vi "MeanderCtrl_Dynamic,StageRefs.vi"(0 "QueuesRef":T1, 1 "MotionStageRefs":refnum<queue>, 2 "AppsRef":refnum<queue>, 3 "subprog_Ref":refnum<vi>, 7 "Params.":variant, 9 "Laser_Ctrl":bool, 11 "error in":errorcluster, 12 "HighSpeed":dbl=5.0, 13 "LowSpeed":dbl=0.1) -> (6 "Interupted":bool, 15 "error out":errorcluster)   [LabVIEW 2013]
uses:
  ControlDef/QueueRefs.ctl
  ControlDef/LaserCtrl_Method.ctl
  ControlDef/States-AToF.ctl
  <instrlib>/AnalogDiscSDKLv/VIs/DWF_CtrlQueue.ctl
  <instrlib>/AnalogDiscSDKLv/VIs/DWF_State.ctl
  <instrlib>/ESP300/Public/Data/ESP300_State.ctl
  <instrlib>/DG535/Command/DG535_States.ctl
  Hardware/BNC(QuantumComposers)/BNC_States.ctl
  Hardware/FemtoLaser(Legacy)/Laser_Status.ctl
  Hardware/DAQmx(Legacy)/DAQmx_Status.ctl
  ControlDef/Signal.ctl
  ProcessMethods/SignalAverager/ProcessStates.ctl
  Files/WriterState.ctl
  Files/Signal_Segment.ctl
  ControlDef/ProcessingMode.ctl
  Hardware/EPM2000(Legacy)/EPM2K_Status.ctl
  <instrlib>/AnalogDiscSDKLv/VIs/DWF_Signal.ctl
  Apps_static/MeanderLoopState.ctl
  Apps_static/ScanParams_SingleLine.ctl
  <instrlib>/ESP300/Public/Data/ESP30x_Data.ctl
  <vilib>/Utility/error.llb/DialogType.ctl
  ControlDef/PauseMeander.vi
  <instrlib>/ESP300/ESP300.lvlib
  <instrlib>/DG535/SRS_DG535_Lib.lvlib
  <userlib>/Utility/ErrorLog_lib.lvlib
  <instrlib>/AnalogDiscSDKLv/AnalogDiscSDKLv.lvlib
panel:
  in  "TotalScan":i32
  out "timed out?":bool
  out "Core_iter.":i32
  out "Scanned Lines":i32
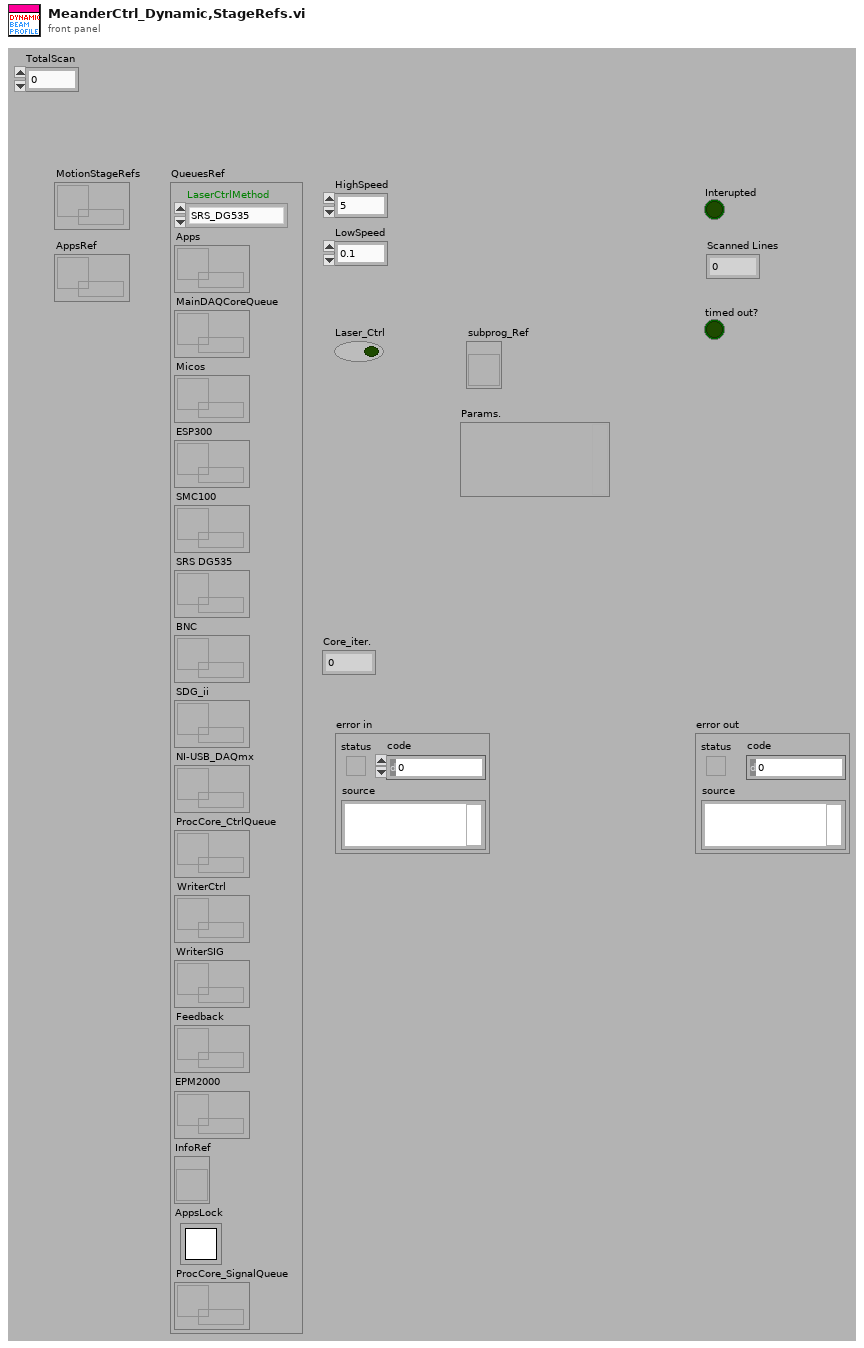
[diagram p1: front panel]
types:
  T1 = typedef "QueueRefs.ctl" = cluster{"LaserCtrlMethod":T2, "Apps":refnum<queue>, "MainDAQCoreQueue":refnum<queue>, "Micos":refnum<queue>, "ESP300":refnum<queue>, "SMC100":refnum<queue>, "SRS DG535":refnum<queue>, "BNC":refnum<queue>, "SDG_ii":refnum<queue>, "NI-USB_DAQmx":refnum<queue>, "ProcCore_CtrlQueue":refnum<queue>, "WriterCtrl":refnum<queue>, "WriterSIG":refnum<queue>, "Feedback":refnum<queue>, "EPM2000":refnum<queue>, "InfoRef":refnum<vi>, "AppsLock":T3, "ProcCore_SignalQueue":refnum<queue>}
  T2 = typedef "LaserCtrl_Method.ctl" = enum16{"SRS_DG535", "BNC", "SDG_II"}
  T3 = typedef "Semaphore RefNum" = refnum<k1>
  T4 = typedef "States-AToF.ctl" = enum16{"Initialize", "Idle", "CalcMzArray", "Meander_SGL_MCS", "Meander_MCS", "CleanSurface", "Meander_Npt", "Meander_SGL_Npt", "KnifeEdgeExpt", "KnifeEdgeExpt_Npt", "Imaging_Micos", "Imaging_ESP", "DepthProfiling", "Set_2PulseDelay", "DelayScan", "PeakSearch", "ExportOrigin", "Save Settings", "Load Settings", "Save as Default", "Load Default", "EnergyCalibration", "Quit", "Interrupted_Stop", "Quit_SubProgram", "StepMove_Joystick", "ContMove_Joystick", "Stop_Joystick", "Check_AppsLock", "Return_Status", "DepthProfile_RT", "UpdateInstruStates", "InstruOptimizer_static", "InstruOptimizer_dynamic", "DepthProfiling(3D)"}
  T5 = typedef "ScanParams_SingleLine.ctl" = cluster{"Line Start":dbl[], "Line End":dbl[], "HighSpeed":dbl, "ScanSpeed":dbl, "KeepStill(ms)":u32, "InstruParams":dbl[]}
  T6 = typedef "MeanderLoopState.ctl" = enum16{"Pre-Start", "Send-loginfo", "SetHighVelocity", "MoveToLineStart", "SetSecondaryParams", "WaitStartReady", "UpdateStartPosition", "StartOfLine", "SetLowVelocity", "MoveToLineEnd", "StartLaser_move", "WaitScanFinish", "StartLaser_still", "KeepStill", "StopLaser", "EndOfLine", "CheckPause", "Exit", "RestoreVelocity", "Pause", "Quit"}
  T7 = typedef "ESP300.lvlib/ESP300_State.ctl" = cluster{"State":enum16{"Initialize", "SetDefaultConfig", "Close", "Quit", "Identify", "MoveAbs", "MoveAbs_all", "MoveRel", "MoveRel_all", "STOP", "Origin/Home", "WaitStop", "QueryStatus", "UpdateXPos", "UpdateAll", "SetVelocity", "SetAcceleration", "ClearErr", "LogMessage", "MotorEnable(1)", "EnableAxis", "JoyStick", "GetVelocity", "GetAcceleration", "SendCmd", "SetSoftLimits", "Beep", "_SettingReturn", "SoftReset"}, "Params.":variant}
  T8 = typedef "ESP300.lvlib/ESP30x_Data.ctl" = cluster{"Position":dbl[], "Velocity":dbl[], "Acceleration":dbl[], "Moving":bool, "Simulation":bool, "tickcount_mov":u32, "tickcount_pos":u32, "NumOfAxis":i32, "Initialized":bool, "CommPort":refnum<visa-resource-name>, "Range":dbl[][], "Serial Configuration":cluster{"Baud Rate":u32, "Parity":u16, "Data Bits":u16, "Stop Bits":u16, "Flow Control":u16}, "MotorDisabled":refnum<vi>}
  T9 = typedef "Signal.ctl" = cluster{"Command":T10, "Params":variant}
  T10 = typedef "ProcessStates.ctl" = enum16{"Initialize", "Normal", "Display", "Write2Buffer", "CalcMzArray", "StartSave", "StopSave", "ConfigChanged", "EndOfLine", "SetFilterParams", "SetGraphsEnable", "SetAcquisitionParams", "ChangeDisplayIncrement", "ChangeRepRate", "SetWriterRef", "Quit", "StartOfLine"}
  T11 = typedef "Laser_Status.ctl" = cluster{"State":enum16{"Initialize", "Idle/Update", "Configure", "Turn On", "Tun OFF", "Continuous", "Single Shot", "ManualTrigger", "Close", "Quit"}, "Parameter":dbl}
  T12 = typedef "BNC_States.ctl" = cluster{"State":enum16{"Initialize", "Set System", "Set C-Input", "Set C-Mode", "Set C-Output", "Set C-Enable", "Manl_Trig", "Run", "Stop", "Query C Number", "Close", "Quit"}, "Para.":variant}
  T13 = typedef "SRS_DG535_Lib.lvlib/DG535_States.ctl" = cluster{"State":enum16{"Initialize", "Set Trigger", "Set Output", "Set Delay", "Manl_Trig", "Run", "Stop", "Close", "Quit"}, "Para.":variant}
  T14 = enum16{"Pre-Start", "Send-loginfo", "SetHighVelocity", "MoveToLineStart", "WaitStartReady", "UpdateStartPosition", "StartOfLine", "SetLowVelocity", "MoveToLineEnd", "StartLaser", "WaitScanFinish", "StopLaser", "EndOfLine", "CheckPause", "Exit", "RestoreHighVelocity", "Pause"}
  T15 = cluster{"Line Start[0]":dbl, "Line Start[1]":dbl, "Line Start[2]":dbl}
  T16 = cluster{"Line End[0]":dbl, "Line End[1]":dbl, "Line End[2]":dbl}
  T17 = typedef "DialogType.ctl" = u16
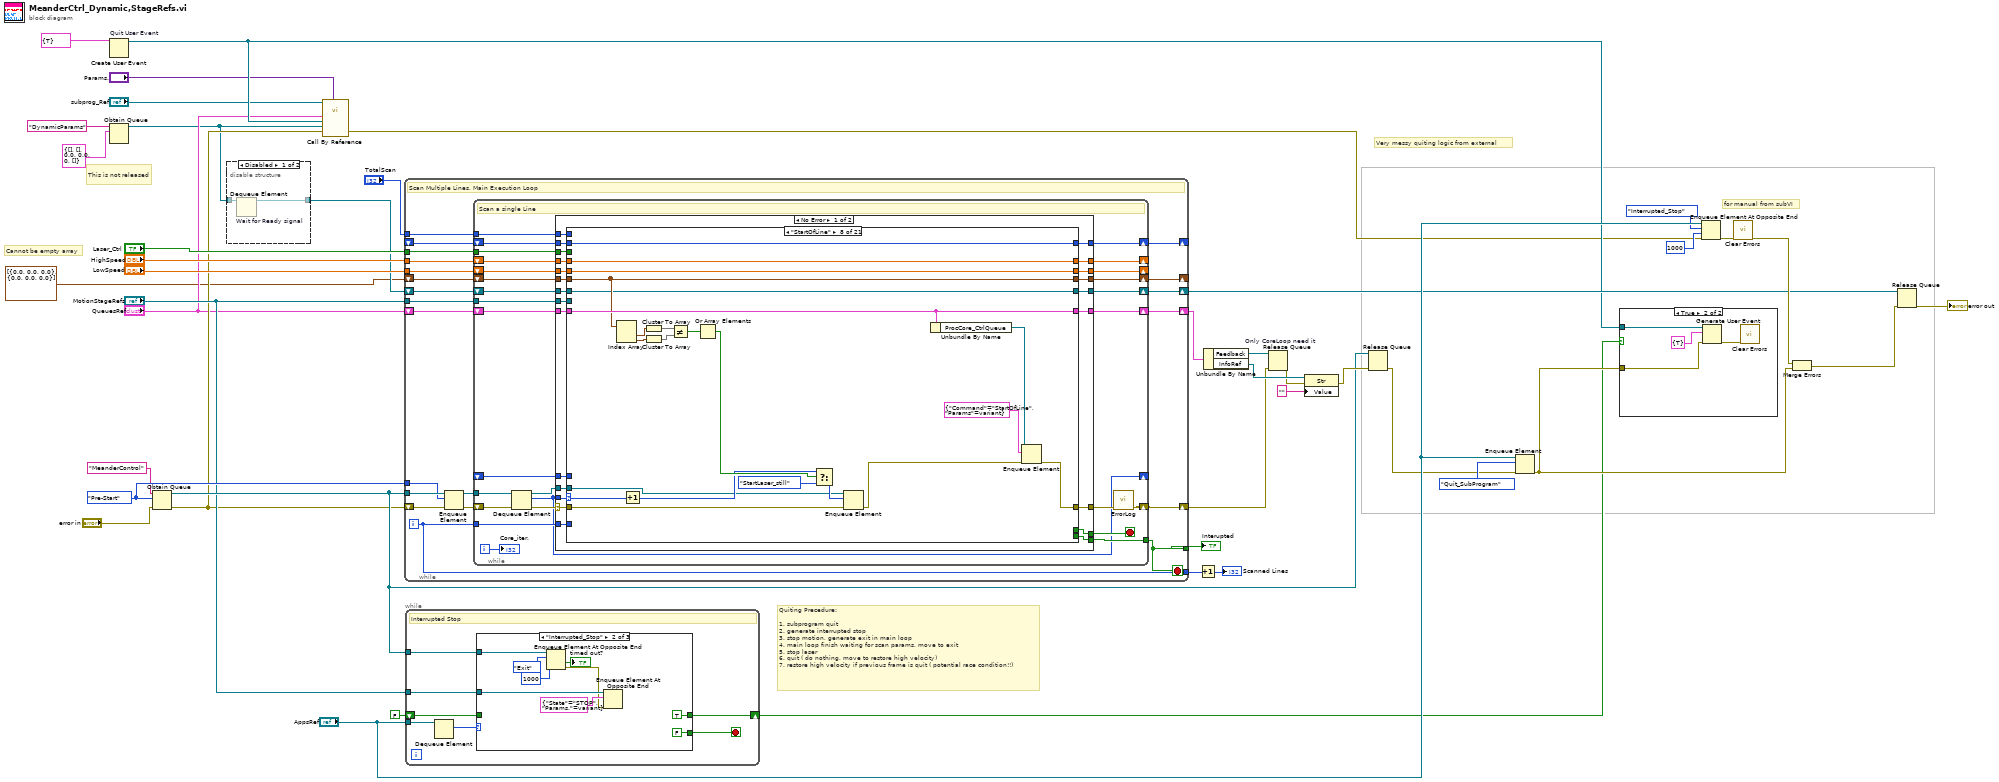
[diagram p0: block diagram]
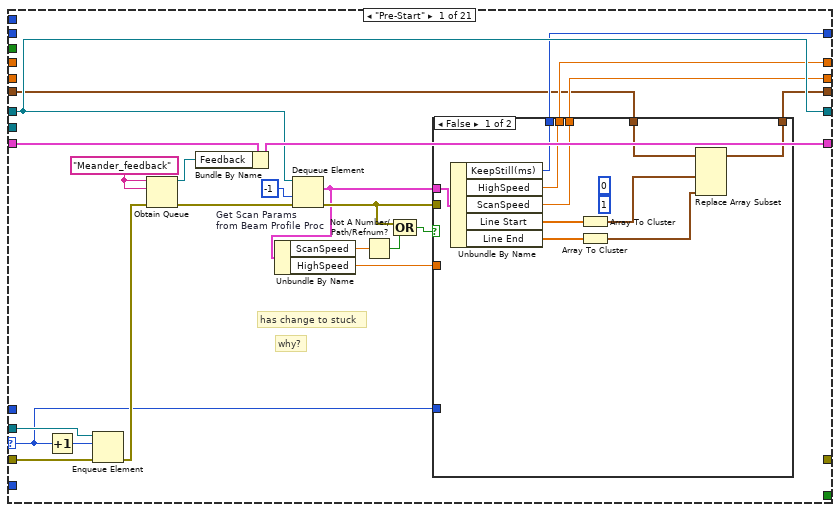
[diagram p2: hidden frame]
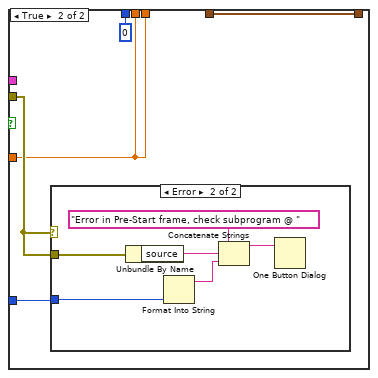
[diagram p3: hidden frame]
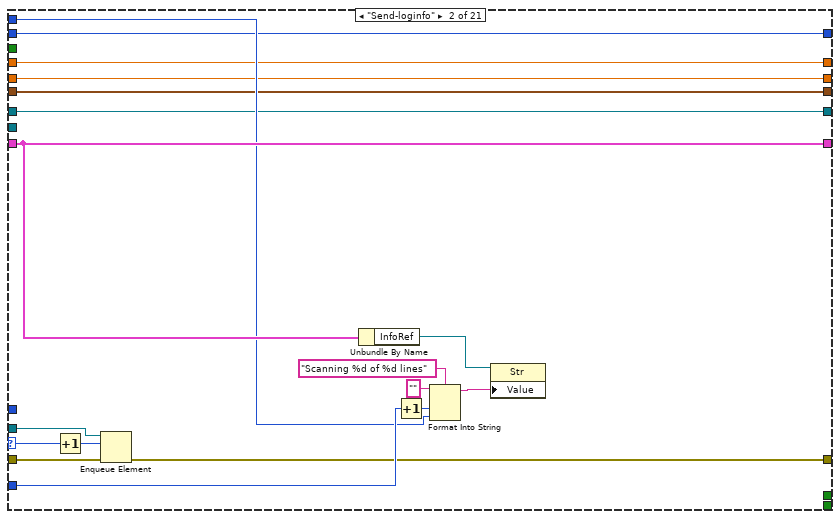
[diagram p5: hidden frame]
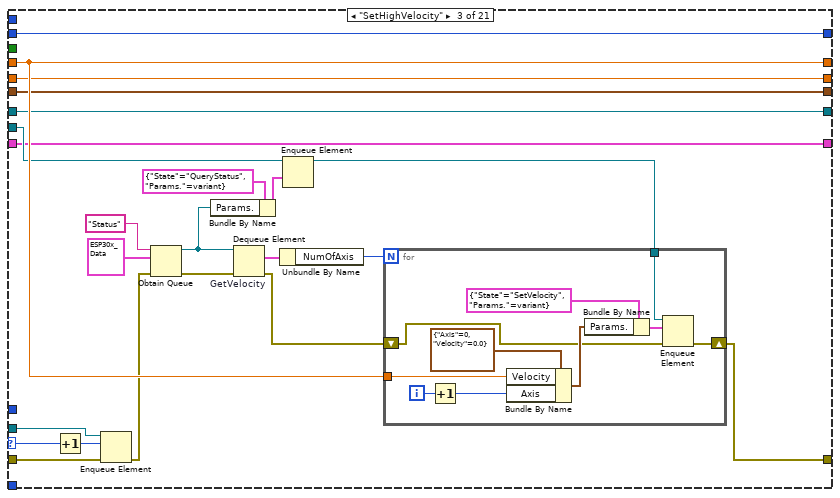
[diagram p6: hidden frame]
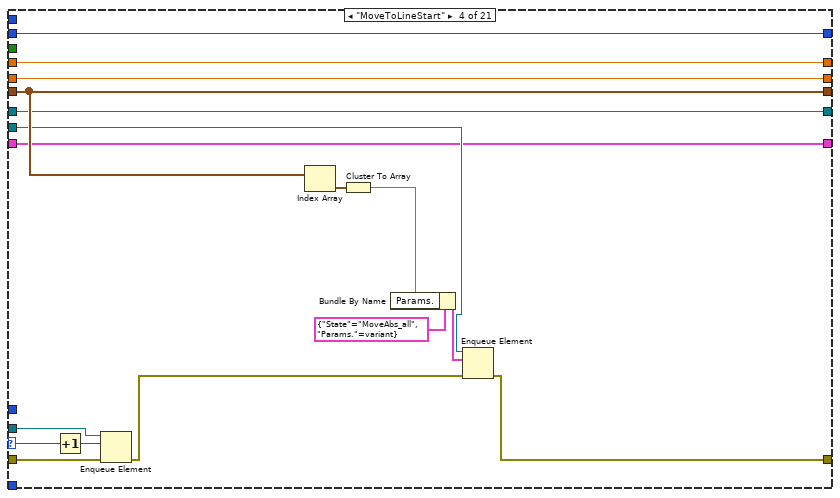
[diagram p7: hidden frame]
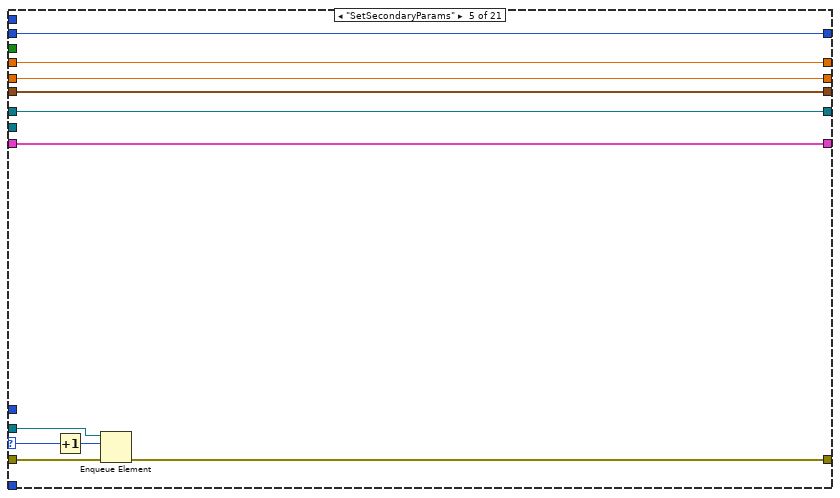
[diagram p8: hidden frame]
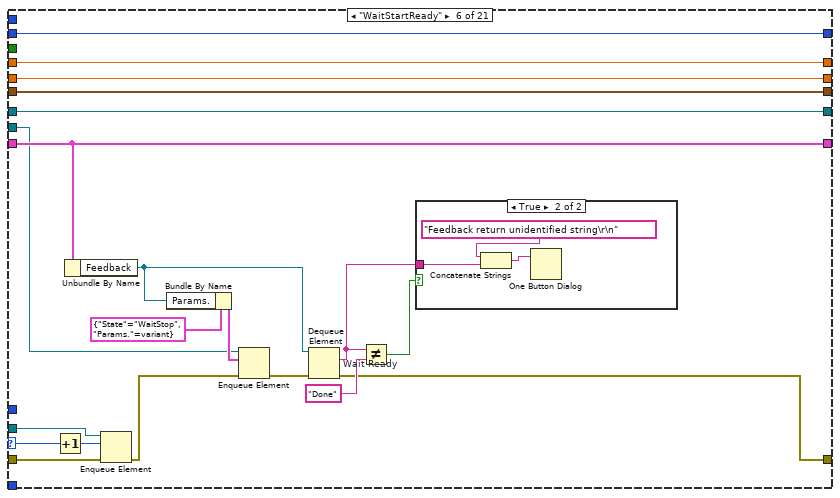
[diagram p9: hidden frame]
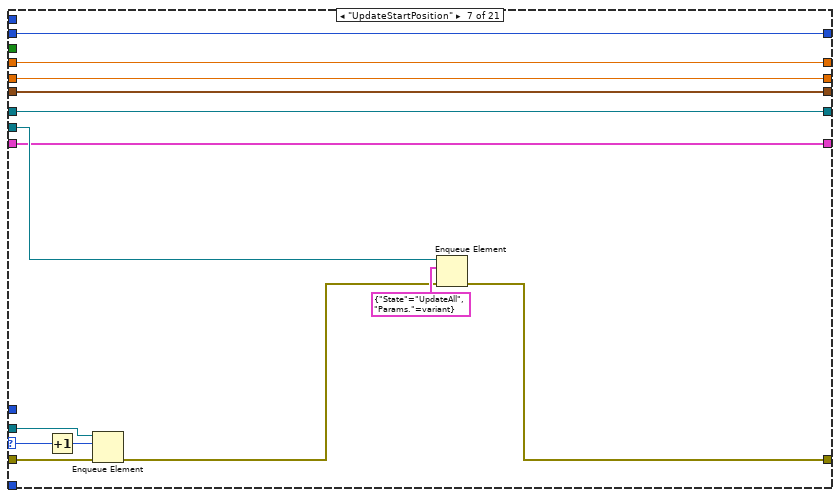
[diagram p11: hidden frame]
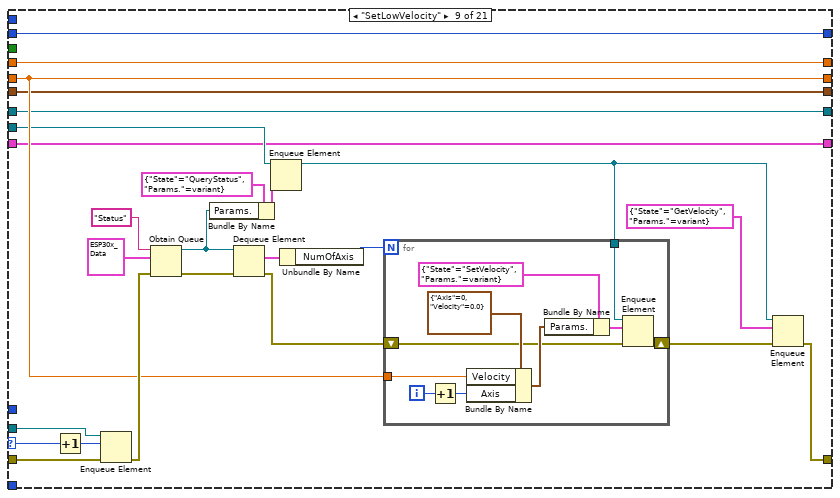
[diagram p12: hidden frame]
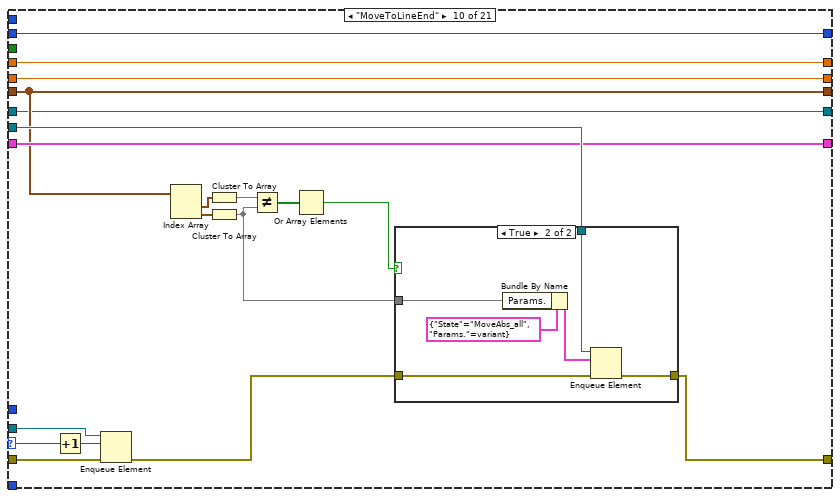
[diagram p13: hidden frame]
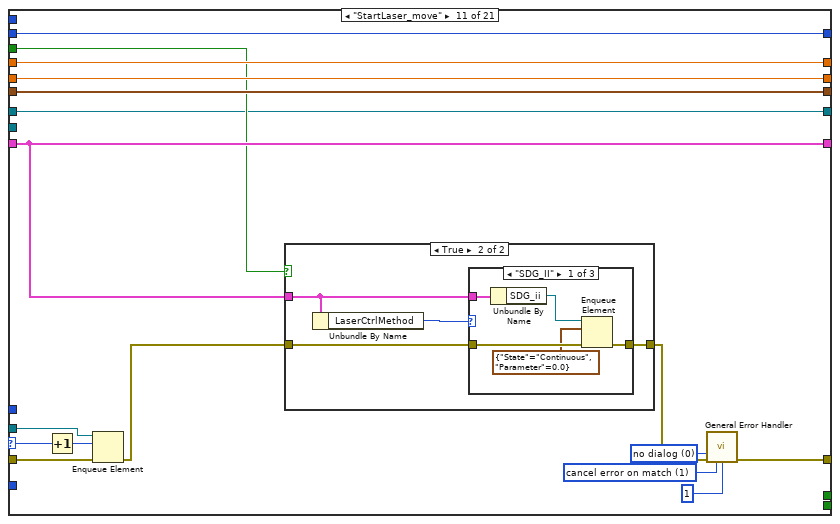
[diagram p15: hidden frame]
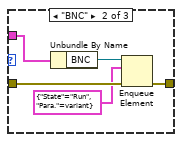
[diagram p17: hidden frame]
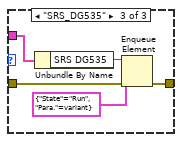
[diagram p18: hidden frame]
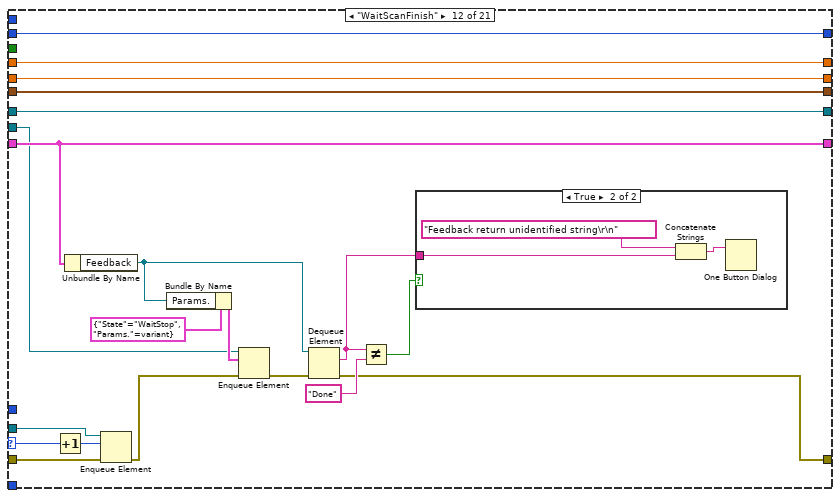
[diagram p19: hidden frame]
diagram:
  w38 = MeanderLoopState."Pre-Start"
  # "Cannot be empty array"
  # "Quiting Precedure:\n\n1. subprogram quit\n2. generate interrupted stop\n3. stop motion, generate exit in main loop\n4. main loop finish waiting for scan params, move to exit \n5. stop laser\n6. quit ( do nothing, move to restore high velocity)\n7. restore high velocity if previous frame is quit ( potential race condition!!)"
  # "Very messy quiting logic from external"
  # "This is not released"
  # "for manual from subVI"
  n1 = Create User Event "Quit User Event"(user event datatype=cluster{"Quit":bool} {"Quit"=TRUE} ("Quit")) -> (user event=w10:refnum<user-event>)  [unwired: 1 in, 1 out]
  n2 = Obtain Queue(name (unnamed)="DynamicParams", element data type=T5 {"Line Start"=[], "Line End"=[], "HighSpeed"=0.0, "ScanSpeed"=0.0, "KeepStill(ms)"=0, "InstruParams"=[]}) -> (queue out=w3:refnum<queue>)  [unwired: 3 in, 2 out]
  n3 = Obtain Queue(name (unnamed)="MeanderControl", element data type=w38, error in (no error)="error in") -> (queue out=w23:refnum<queue>, error out=w9:errorcluster)  [unwired: 2 in, 1 out]
  n4 = disable-structure shown="Disabled" {
    disable-tunnel: w3 -> [w46 w47]
    disable-tunnel: [w45 w47] -> w4
    frame Disabled {
      n5 = Dequeue Element "Wait for Ready signal"(queue=w46) -> (queue out=w45:refnum<queue>)  [unwired: 2 in, 3 out]
    }
    frame Enabled {
    }
  }
  n6 = call-by-ref "?"(reference="subprog_Ref", "Params."="Params.", "error in (no error)"=w9, "Dynamic Params In"=w3, "Quit_UserEvent"=w10, "ControlQueueRef"="QueuesRef") -> ("error out"=w8:errorcluster)  [unwired: 6 in, 3 out]
  n7 = while {
    tunnel: "MotionStageRefs" -> [w67]
    tunnel: w23 -> [w63]
    tunnel: "Laser_Ctrl" -> [w62]
    tunnel: [w61] -> w42
    shift-right: [w60] -> w29
    shift-left: w9 -> [w59]
    tunnel: [w58] -> w39
    tunnel: w38 -> [w56]
    shift-right: [w55] -> w31
    shift-left: "QueuesRef" -> [w66]
    tunnel: "HighSpeed" -> [w64]
    tunnel: "LowSpeed" -> [w65]
    shift-right: [w50] -> w16
    shift-left: w4 -> [w54]
    shift-right: [w49] -> _
    shift-left: _ -> [w53]
    tunnel: "TotalScan" -> [w48]
    shift-right: [w51] -> _
    shift-left: cluster{dbl, dbl, dbl}[] [{0.0, 0.0, 0.0}, {0.0, 0.0, 0.0}] ("start/end points") -> [w52]
    i -> [w61]
    stop <- w58 stop-if-true
    # "Scan Multiple Lines, Main Execution Loop"
    n8 = Enqueue Element(queue=w63, element=w56) -> (queue out=w57:refnum<queue>)  [unwired: 2 in, 2 out]
    n9 = while {
      tunnel: w67 -> [w94]
      tunnel: w57 -> [w90]
      tunnel: w61 -> [w88]
      shift-right: [w68] -> w60
      shift-left: w59 -> [w71]
      tunnel: w62 -> [w85]
      shift-right: [w69] -> _
      shift-left: _ -> [w84]
      tunnel: [w83] -> w58
      tunnel: w48 -> [w82]
      shift-right: [w81] -> w55
      shift-left: w66 -> [w93]
      shift-right: [w79] -> _
      shift-left: w64 -> [w91]
      shift-right: [w80] -> _
      shift-left: w65 -> [w92]
      shift-right: [w75] -> w49
      shift-left: w53 -> [w77]
      shift-right: [w76] -> w51
      shift-left: w52 -> [w74]
      shift-right: [w70] -> w50
      shift-left: w54 -> [w78]
      i -> [w73]
      stop <- w89 stop-if-true
      # "Scan a single Line"
      n10 = Dequeue Element(queue=w90, error in (no error)=w71) -> (queue out=w87:refnum<queue>, element=w69:T6, error out=w72:errorcluster)  [unwired: 1 in, 1 out]
      n11 = case shown="No Error" w72 {
        selector: w72 -> [w96 w671]
        tunnel: w94 -> [w117 _]
        tunnel: w93 -> [w116 w675]
        tunnel: w92 -> [w115 w674]
        tunnel: w91 -> [w114 w673]
        tunnel: [w113 _] -> w89
        tunnel: w88 -> [w112 _]
        tunnel: w87 -> [w111 _]
        tunnel: [w110 _] -> w86
        tunnel: w85 -> [w109 _]
        tunnel: w69 -> [w108 _]
        tunnel: w84 -> [w107 w666]
        tunnel: [w106 _] -> w83
        tunnel: w82 -> [w105 _]
        tunnel: [w104 w675] -> w81
        tunnel: [w103 w674] -> w80
        tunnel: [w102 w673] -> w79
        tunnel: w78 -> [w101 w669]
        tunnel: w77 -> [w100 w672]
        tunnel: [w99 w665] -> w76
        tunnel: [w98 w672] -> w75
        tunnel: w74 -> [w97 w665]
        tunnel: [w95 w669] -> w70
        frame No Error {
          n12 = case shown="\"StartOfLine\"" w108 {
            selector: w108 -> [w119 w179 w202 w229 w240 w260 w277 w282 w324 w353 w377 w417 w439 w470 w488 _ _ _ _ _ _]
            tunnel: w117 -> [_ _ w185 w218 _ w246 w272 _ w310 w347 _ w403 _ _ _ _ _ w562 w579 w609 _]
            tunnel: w116 -> [w137 w174 w184 w217 w234 w258 w269 w299 w309 w346 w368 w415 w429 w468 w484 w519 w527 w556 w578 w608 w637]
            tunnel: w115 -> [_ w165 w183 w215 w232 w244 w267 w295 w311 w344 w372 w401 w434 w463 w480 w514 w525 w554 w577 w607 w635]
            tunnel: w114 -> [_ w166 w198 w216 w233 w245 w268 w296 w307 w345 w373 w402 w435 w464 w481 w515 w526 w555 w591 w621 w636]
            tunnel: [_ _ _ _ _ _ _ _ _ _ _ _ _ _ _ _ TRUE FALSE _ w602 _] -> w113
            tunnel: w112 -> [_ w172 _ _ _ _ _ _ _ _ _ _ _ _ _ _ _ _ _ _ _]
            tunnel: w111 -> [w138 w171 w200 w227 w238 w257 w275 w283 w322 w351 w375 w414 w437 w467 w486 w521 w530 w547 w572 _ w641]
            tunnel: w96 -> [w139 w170 w199 w226 w237 w256 w274 w284 w321 w350 w374 w413 w436 w466 w485 w520 w531 w563 w573 w603 w644]
            tunnel: [_ w169 w187 w219 w235 w247 w270 w297 w302 w348 w365 w404 w423 w465 w473 w516 w528 _ w581 w611 w643] -> w110
            tunnel: w97 -> [w128 w164 w182 w223 w236 w243 w266 w281 w306 w338 w371 w400 w433 w462 w479 w513 w524 w553 w576 w606 w634]
            tunnel: w109 -> [_ _ _ _ _ _ _ _ _ _ w367 _ w430 _ w483 _ _ _ _ _ _]
            tunnel: w107 -> [_ _ _ _ _ _ _ _ _ _ _ _ _ _ _ _ _ _ _ _ _]
            tunnel: [_ _ _ _ _ _ _ _ _ _ _ _ _ _ _ _ w529 _ _ w602 _] -> w106
            tunnel: w105 -> [_ w167 _ _ _ _ _ _ _ _ _ _ _ _ _ _ _ _ _ _ _]
            tunnel: [w136 w174 w184 w217 w234 w258 w269 w299 w309 w346 w368 w415 w429 w468 w484 w519 w527 w556 w578 w608 w637] -> w104
            tunnel: [w131 w165 w183 w215 w232 w244 w267 w295 w311 w344 w372 w401 w434 w463 w480 w514 w525 w554 w577 w607 w635] -> w103
            tunnel: [w132 w166 w198 w216 w233 w245 w268 w296 w307 w345 w373 w402 w435 w464 w481 w515 w526 w555 w591 w621 w636] -> w102
            tunnel: w101 -> [w133 w162 w180 w213 w230 w241 w264 w278 w300 w335 w361 w398 w421 w460 w472 w510 w522 w548 w574 w604 w632]
            tunnel: w100 -> [_ w163 w181 w214 w231 w242 w265 w294 w305 w343 w370 w399 w431 w461 w478 w512 w523 w552 w575 w605 w633]
            tunnel: [w127 w164 w182 w223 w236 w243 w266 w281 w306 w338 w371 w400 w433 w462 w479 w513 w524 w553 w576 w606 w634] -> w99
            tunnel: [w130 w163 w181 w214 w231 w242 w265 w294 w305 w343 w370 w399 w431 w461 w478 w512 w523 w552 w575 w605 w633] -> w98
            tunnel: [w133 w162 w180 w213 w230 w241 w264 w278 w300 w335 w361 w398 w421 w460 w472 w510 w522 w548 w574 w604 w632] -> w95
            frame "Pre-Start" {
              w134 = "Meander_feedback" ("name (unnamed)")
              # "why?"
              # "has change to stuck"
              n13 = Increment(x=w119) -> (x+1=w140:T6)
              n14 = Enqueue Element(queue=w138, element=w140, error in (no error)=w139) -> (error out=w125:errorcluster)  [unwired: 1 in, 2 out]
              n15 = Obtain Queue(name (unnamed)=w134, element data type=w134, error in (no error)=w125) -> (queue out=w135:refnum<queue>, error out=w129:errorcluster)  [unwired: 2 in, 1 out]
              n16 = Bundle By Name(cluster=w137, "Feedback"=w135) -> (w136:T1)
              n17 = Dequeue Element "Get Scan Params\nfrom Beam Profile Proc"(queue=w133, timeout in ms (-1)=-1, error in (no error)=w129) -> (element=w122:T5, error out=w123:errorcluster)  [unwired: 2 out]
              n18 = Unbundle By Name(w122) -> ("ScanSpeed"=w121:dbl, "HighSpeed"=w118:dbl)
              n19 = Not A Number/Path/Refnum?(number/path/refnum=w121) -> (NaN/Path/Refnum?=w120:bool)
              n20 = Compound Arithmetic op=OR(w123, w120) -> (w124:bool)
              n21 = case shown="False" w124 {
                tunnel: w122 -> [w150 _]
                tunnel: [w149 w153] -> w132
                tunnel: [w148 w153] -> w131
                tunnel: [w147 u32 0 ("KeepStill(ms)")] -> w130
                tunnel: w128 -> [w144 w151]
                tunnel: [w143 w151] -> w127
                tunnel: w123 -> [_ w155]
                tunnel: w119 -> [_ w154]
                tunnel: w118 -> [_ w153]
                frame False {
                  (unwired) 1
                  (unwired) 0
                  n22 = Unbundle By Name(w150) -> ("KeepStill(ms)"=w147:u32, "HighSpeed"=w149:dbl, "ScanSpeed"=w148:dbl, "Line Start"=w146:dbl[], "Line End"=w145:dbl[])
                  n23 = Array To Cluster(array=w146) -> (cluster=w142:T15)
                  n24 = Array To Cluster(array=w145) -> (cluster=w141:T16)
                  n25 = Replace Array Subset(array=w144, new element #1=w142, new element #2=w141) -> (w143:cluster{dbl, dbl, dbl}[])  [unwired: 2 in]
                }
                frame True {
                  n26 = case shown="Error" w155 {
                    tunnel: w155 -> [_ w158]
                    tunnel: w154 -> [_ w157]
                    frame No Error {
                    }
                    frame Error {
                      n27 = Unbundle By Name(w158) -> ("source"=w159:string)
                      n28 = Format Into String(w157) -> (resulting string=w156:string)  [unwired: 3 in, 1 out]
                      n29 = Concatenate Strings("Error in Pre-Start frame, check subprogram @ " ("message"), w159, w156) -> (w161:string)
                      n30 = One Button Dialog(message=w161) -> ()  [unwired: 1 in, 1 out]
                    }
                  }
                }
              }
            }
            frame "Send-loginfo" {
              n31 = Increment(x=w179) -> (x+1=w178:T6)
              n32 = Enqueue Element(queue=w171, element=w178, error in (no error)=w170) -> (error out=w169:errorcluster)  [unwired: 1 in, 2 out]
              n33 = Unbundle By Name(w174) -> ("InfoRef"=w173:refnum<vi>)
              n34 = Increment(x=w172) -> (x+1=w176:i32)
              n35 = Format Into String(format string="Scanning %d of %d lines", initial string="", w176, w167) -> (resulting string=w177:string)  [unwired: 1 in, 1 out]
              n36 = property class="Str"(reference=w173, "Value"=w177) -> ()  [unwired: 1 in, 2 out]
            }
            frame "SetHighVelocity" {
              n37 = Increment(x=w202) -> (x+1=w201:T6)
              n38 = Enqueue Element(queue=w200, element=w201, error in (no error)=w199) -> (error out=w188:errorcluster)  [unwired: 1 in, 2 out]
              n39 = Obtain Queue(name (unnamed)="Status", element data type=T8 {"Position"=[], "Velocity"=[], "Acceleration"=[], "Moving"=FALSE, "Simulation"=FALSE, "tickcount_mov"=0, "tickcount_pos"=0, "NumOfAxis"=0, "Initialized"=FALSE, "CommPort"="", "Range"=[], "Serial Configuration"={"Baud Rate"=0, "Parity"=0, "Data Bits"=0, "Stop Bits"=0, "Flow Control"=0}, "MotorDisabled"=refnum}, error in (no error)=w188) -> (queue out=w193:refnum<queue>, error out=w192:errorcluster)  [unwired: 2 in, 1 out]
              n40 = Bundle By Name(cluster=T7 {"State"=enum."QueryStatus", "Params."=variant} ("element"), "Params."=w193) -> (w194:T7)
              n41 = Dequeue Element "GetVelocity"(queue=w193, error in (no error)=w192) -> (element=w191:T8, error out=w189:errorcluster)  [unwired: 1 in, 2 out]
              n42 = Unbundle By Name(w191) -> ("NumOfAxis"=w190:i32)
              n43 = Enqueue Element(queue=w185, element=w194) -> (queue out=w197:refnum<queue>)  [unwired: 2 in, 2 out]
              n44 = for {
                N: w190 -> [_]
                tunnel: w197 -> [w206]
                tunnel: w198 -> [w205]
                shift-right: [w203] -> w187
                shift-left: w189 -> [w204]
                i -> [w212]
                n45 = Increment(x=w212) -> (x+1=w210:i32)
                n46 = Bundle By Name(cluster=cluster{"Axis":i32, "Velocity":dbl} {"Axis"=0, "Velocity"=0.0}, "Velocity"=w205, "Axis"=w210) -> (w207:cluster{"Axis":i32, "Velocity":dbl})
                n47 = Bundle By Name(cluster=T7 {"State"=enum."SetVelocity", "Params."=variant} ("element"), "Params."=w207) -> (w209:T7)
                n48 = Enqueue Element(queue=w206, element=w209, error in (no error)=w204) -> (error out=w203:errorcluster)  [unwired: 1 in, 2 out]
              }
            }
            frame "MoveToLineStart" {
              n49 = Increment(x=w229) -> (x+1=w228:T6)
              n50 = Enqueue Element(queue=w227, element=w228, error in (no error)=w226) -> (error out=w220:errorcluster)  [unwired: 1 in, 2 out]
              n51 = Index Array(array=w223) -> (element=w222:cluster{dbl, dbl, dbl})  [unwired: 1 in]
              n52 = Cluster To Array(cluster=w222) -> (array=w221:dbl[])
              n53 = Bundle By Name(cluster=T7 {"State"=enum."MoveAbs_all", "Params."=variant} ("element"), "Params."=w221) -> (w224:T7)
              n54 = Enqueue Element(queue=w218, element=w224, error in (no error)=w220) -> (error out=w219:errorcluster)  [unwired: 1 in, 2 out]
            }
            frame "SetSecondaryParams" {
              n55 = Increment(x=w240) -> (x+1=w239:T6)
              n56 = Enqueue Element(queue=w238, element=w239, error in (no error)=w237) -> (error out=w235:errorcluster)  [unwired: 1 in, 2 out]
            }
            frame "WaitStartReady" {
              n57 = Increment(x=w260) -> (x+1=w259:T6)
              n58 = Unbundle By Name(w258) -> ("Feedback"=w251:refnum<queue>)
              n59 = Enqueue Element(queue=w257, element=w259, error in (no error)=w256) -> (error out=w253:errorcluster)  [unwired: 1 in, 2 out]
              n60 = Bundle By Name(cluster=T7 {"State"=enum."WaitStop", "Params."=variant} ("element"), "Params."=w251) -> (w254:T7)
              n61 = Enqueue Element(queue=w246, element=w254, error in (no error)=w253) -> (error out=w252:errorcluster)  [unwired: 1 in, 2 out]
              n62 = Dequeue Element "Wait Ready"(queue=w251, error in (no error)=w252) -> (element=w248:string, error out=w247:errorcluster)  [unwired: 1 in, 2 out]
              n63 = Not Equal?(x=w248, y="Done" ("element")) -> (x != y?=w249:bool)
              n64 = case shown="True" w249 {
                tunnel: w248 -> [_ w261]
                frame False {
                }
                frame True {
                  n65 = Concatenate Strings("Feedback return unidentified string\r\n" ("message"), w261) -> (w262:string)
                  n66 = One Button Dialog(message=w262) -> ()  [unwired: 1 in, 1 out]
                }
              }
            }
            frame "UpdateStartPosition" {
              n67 = Increment(x=w277) -> (x+1=w276:T6)
              n68 = Enqueue Element(queue=w275, element=w276, error in (no error)=w274) -> (error out=w271:errorcluster)  [unwired: 1 in, 2 out]
              n69 = Enqueue Element(queue=w272, element=T7 {"State"=enum."UpdateAll", "Params."=variant}, error in (no error)=w271) -> (error out=w270:errorcluster)  [unwired: 1 in, 2 out]
            }
            frame "StartOfLine" {
              n70 = Index Array(array=w281) -> (element #1=w287:cluster{dbl, dbl, dbl}, element #2=w286:cluster{dbl, dbl, dbl})  [unwired: 2 in]
              n71 = Increment(x=w282) -> (x+1=w291:T6)
              n72 = Cluster To Array(cluster=w287) -> (array=w288:dbl[])
              n73 = Cluster To Array(cluster=w286) -> (array=w289:dbl[])
              n74 = Not Equal?(x=w288, y=w289) -> (x != y?=w290:bool[])
              n75 = Or Array Elements(Boolean array=w290) -> (logical OR=w293:bool)
              n76 = Select(t=w291, s=w293, f=MeanderLoopState."StartLaser_still") -> (s? t:f=w285:T6)
              n77 = Enqueue Element(queue=w283, element=w285, error in (no error)=w284) -> (error out=w280:errorcluster)  [unwired: 1 in, 2 out]
              n78 = Unbundle By Name(w299) -> ("ProcCore_CtrlQueue"=w298:refnum<queue>)
              n79 = Enqueue Element(queue=w298, element=T9 {"Command"=enum."StartOfLine", "Params"=variant}, error in (no error)=w280) -> (error out=w297:errorcluster)  [unwired: 1 in, 2 out]
            }
            frame "SetLowVelocity" {
              n80 = Increment(x=w324) -> (x+1=w323:T6)
              n81 = Enqueue Element(queue=w322, element=w323, error in (no error)=w321) -> (error out=w312:errorcluster)  [unwired: 1 in, 2 out]
              n82 = Obtain Queue(name (unnamed)="Status", element data type=T8 {"Position"=[], "Velocity"=[], "Acceleration"=[], "Moving"=FALSE, "Simulation"=FALSE, "tickcount_mov"=0, "tickcount_pos"=0, "NumOfAxis"=0, "Initialized"=FALSE, "CommPort"="", "Range"=[], "Serial Configuration"={"Baud Rate"=0, "Parity"=0, "Data Bits"=0, "Stop Bits"=0, "Flow Control"=0}, "MotorDisabled"=refnum}, error in (no error)=w312) -> (queue out=w317:refnum<queue>, error out=w316:errorcluster)  [unwired: 2 in, 1 out]
              n83 = Bundle By Name(cluster=T7 {"State"=enum."QueryStatus", "Params."=variant} ("element"), "Params."=w317) -> (w318:T7)
              n84 = Dequeue Element(queue=w317, error in (no error)=w316) -> (element=w315:T8, error out=w313:errorcluster)  [unwired: 1 in, 2 out]
              n85 = Enqueue Element(queue=w310, element=w318) -> (queue out=w301:refnum<queue>)  [unwired: 2 in, 2 out]
              n86 = Unbundle By Name(w315) -> ("NumOfAxis"=w314:i32)
              n87 = for {
                N: w314 -> [_]
                tunnel: w301 -> [w328]
                tunnel: w311 -> [w327]
                shift-right: [w325] -> w303
                shift-left: w313 -> [w326]
                i -> [w334]
                n88 = Increment(x=w334) -> (x+1=w332:i32)
                n89 = Bundle By Name(cluster=cluster{"Axis":i32, "Velocity":dbl} {"Axis"=0, "Velocity"=0.0}, "Velocity"=w327, "Axis"=w332) -> (w329:cluster{"Axis":i32, "Velocity":dbl})
                n90 = Bundle By Name(cluster=T7 {"State"=enum."SetVelocity", "Params."=variant} ("element"), "Params."=w329) -> (w331:T7)
                n91 = Enqueue Element(queue=w328, element=w331, error in (no error)=w326) -> (error out=w325:errorcluster)  [unwired: 1 in, 2 out]
              }
              n92 = Enqueue Element(queue=w301, element=T7 {"State"=enum."GetVelocity", "Params."=variant}, error in (no error)=w303) -> (error out=w302:errorcluster)  [unwired: 1 in, 2 out]
            }
            frame "MoveToLineEnd" {
              n93 = Increment(x=w353) -> (x+1=w352:T6)
              n94 = Enqueue Element(queue=w351, element=w352, error in (no error)=w350) -> (error out=w349:errorcluster)  [unwired: 1 in, 2 out]
              n95 = Index Array(array=w338) -> (element #1=w340:cluster{dbl, dbl, dbl}, element #2=w339:cluster{dbl, dbl, dbl})  [unwired: 2 in]
              n96 = Cluster To Array(cluster=w340) -> (array=w341:dbl[])
              n97 = Cluster To Array(cluster=w339) -> (array=w337:dbl[])
              n98 = Not Equal?(x=w341, y=w337) -> (x != y?=w342:bool[])
              n99 = Or Array Elements(Boolean array=w342) -> (logical OR=w336:bool)
              n100 = case shown="True" w336 {
                tunnel: w349 -> [w354 w358]
                tunnel: [w354 w357] -> w348
                tunnel: w347 -> [_ w356]
                tunnel: w337 -> [_ w355]
                frame False {
                }
                frame True {
                  n101 = Bundle By Name(cluster=T7 {"State"=enum."MoveAbs_all", "Params."=variant} ("element"), "Params."=w355) -> (w359:T7)
                  n102 = Enqueue Element(queue=w356, element=w359, error in (no error)=w358) -> (error out=w357:errorcluster)  [unwired: 1 in, 2 out]
                }
              }
            }
            frame "StartLaser_move" {
              w362 = T17 0 items=["no dialog", "OK message", "continue or stop message", "OK message + warnings", "continue/stop + warnings"] ("type of dialog (OK msg:1)")
              w364 = 1 items=["no exception", "cancel error on match", "set error on match"] ("[exception action] (none:0)")
              n103 = Increment(x=w377) -> (x+1=w376:T6)
              n104 = Enqueue Element(queue=w375, element=w376, error in (no error)=w374) -> (error out=w369:errorcluster)  [unwired: 1 in, 2 out]
              n105 = case shown="True" w367 {
                tunnel: [w378 w382] -> w366
                tunnel: w369 -> [w378 w381]
                tunnel: w368 -> [_ w380]
                frame False {
                }
                frame True {
                  n106 = Unbundle By Name(w380) -> ("LaserCtrlMethod"=w379:T2)
                  n107 = case shown="\"SDG_II\"" w379 {
                    tunnel: [w387 w392 w397] -> w382
                    tunnel: w381 -> [w386 w391 w396]
                    tunnel: w380 -> [w384 w390 w395]
                    frame "SDG_II" {
                      n108 = Unbundle By Name(w384) -> ("SDG_ii"=w383:refnum<queue>)
                      n109 = Enqueue Element(queue=w383, element=T11 {"State"=enum."Continuous", "Parameter"=0.0}, error in (no error)=w386) -> (error out=w387:errorcluster)  [unwired: 1 in, 2 out]
                    }
                    frame "BNC" {
                      n110 = Unbundle By Name(w390) -> ("BNC"=w389:refnum<queue>)
                      n111 = Enqueue Element(queue=w389, element=T12 {"State"=enum."Run", "Para."=variant}, error in (no error)=w391) -> (error out=w392:errorcluster)  [unwired: 1 in, 2 out]
                    }
                    frame "SRS_DG535" {
                      n112 = Unbundle By Name(w395) -> ("SRS DG535"=w394:refnum<queue>)
                      n113 = Enqueue Element(queue=w394, element=T13 {"State"=enum."Run", "Para."=variant}, error in (no error)=w396) -> (error out=w397:errorcluster)  [unwired: 1 in, 2 out]
                    }
                  }
                }
              }
              n114 = call <vilib>:"General Error Handler.vi"("type of dialog (OK msg:1)"=w362, "error in (no error)"=w366, "[exception action] (none:0)"=w364, "[exception code]"=1) -> ("error out"=w365:errorcluster)  [unwired: 7 in, 4 out]
            }
            frame "WaitScanFinish" {
              n115 = Increment(x=w417) -> (x+1=w416:T6)
              n116 = Unbundle By Name(w415) -> ("Feedback"=w408:refnum<queue>)
              n117 = Enqueue Element(queue=w414, element=w416, error in (no error)=w413) -> (error out=w410:errorcluster)  [unwired: 1 in, 2 out]
              n118 = Bundle By Name(cluster=T7 {"State"=enum."WaitStop", "Params."=variant} ("element"), "Params."=w408) -> (w411:T7)
              n119 = Enqueue Element(queue=w403, element=w411, error in (no error)=w410) -> (error out=w409:errorcluster)  [unwired: 1 in, 2 out]
              n120 = Dequeue Element(queue=w408, error in (no error)=w409) -> (element=w405:string, error out=w404:errorcluster)  [unwired: 1 in, 2 out]
              n121 = Not Equal?(x=w405, y="Done" ("element")) -> (x != y?=w406:bool)
              n122 = case shown="True" w406 {
                tunnel: w405 -> [_ w418]
                frame False {
                }
                frame True {
                  n123 = Concatenate Strings("Feedback return unidentified string\r\n" ("message"), w418) -> (w419:string)
                  n124 = One Button Dialog(message=w419) -> ()  [unwired: 1 in, 1 out]
                }
              }
            }
            frame "StartLaser_still" {
              w424 = T17 0 items=["no dialog", "OK message", "continue or stop message", "OK message + warnings", "continue/stop + warnings"] ("type of dialog (OK msg:1)")
              w426 = 1 items=["no exception", "cancel error on match", "set error on match"] ("[exception action] (none:0)")
              n125 = Increment(x=w439) -> (x+1=w438:T6)
              n126 = Enqueue Element(queue=w437, element=w438, error in (no error)=w436) -> (error out=w427:errorcluster)  [unwired: 1 in, 2 out]
              n127 = Not Equal To 0?(x=w431) -> (x != 0?=w432:bool)
              n128 = And(x=w432, y=w430) -> (x .and. y?=w428:bool)
              n129 = case shown="True" w428 {
                tunnel: [w440 w444] -> w422
                tunnel: w427 -> [w440 w443]
                tunnel: w429 -> [_ w442]
                frame False {
                }
                frame True {
                  n130 = Unbundle By Name(w442) -> ("LaserCtrlMethod"=w441:T2)
                  n131 = case shown="\"BNC\"" w441 {
                    tunnel: [w449 w454 w459] -> w444
                    tunnel: w443 -> [w448 w453 w458]
                    tunnel: w442 -> [w446 w452 w457]
                    frame "SDG_II" {
                      n132 = Unbundle By Name(w446) -> ("SDG_ii"=w445:refnum<queue>)
                      n133 = Enqueue Element(queue=w445, element=T11 {"State"=enum."Continuous", "Parameter"=0.0}, error in (no error)=w448) -> (error out=w449:errorcluster)  [unwired: 1 in, 2 out]
                    }
                    frame "BNC" {
                      n134 = Unbundle By Name(w452) -> ("BNC"=w451:refnum<queue>)
                      n135 = Enqueue Element(queue=w451, element=T12 {"State"=enum."Run", "Para."=variant}, error in (no error)=w453) -> (error out=w454:errorcluster)  [unwired: 1 in, 2 out]
                    }
                    frame "SRS_DG535" {
                      n136 = Unbundle By Name(w457) -> ("SRS DG535"=w456:refnum<queue>)
                      n137 = Enqueue Element(queue=w456, element=T13 {"State"=enum."Run", "Para."=variant}, error in (no error)=w458) -> (error out=w459:errorcluster)  [unwired: 1 in, 2 out]
                    }
                  }
                }
              }
              n138 = call <vilib>:"General Error Handler.vi"("type of dialog (OK msg:1)"=w424, "error in (no error)"=w422, "[exception action] (none:0)"=w426, "[exception code]"=1) -> ("error out"=w423:errorcluster)  [unwired: 7 in, 4 out]
            }
            frame "KeepStill" {
              n139 = Increment(x=w470) -> (x+1=w469:T6)
              n140 = Enqueue Element(queue=w467, element=w469, error in (no error)=w466) -> (error out=w465:errorcluster)  [unwired: 1 in, 2 out]
              n141 = case shown="Default" w461 {
                selector: w461 -> [_ w471]
                frame 0 {
                }
                frame Default {
                  n142 = Wait (ms)(milliseconds to wait=w471) -> ()  [unwired: 1 out]
                }
              }
            }
            frame "StopLaser" {
              w475 = T17 0 items=["no dialog", "OK message", "continue or stop message", "OK message + warnings", "continue/stop + warnings"] ("type of dialog (OK msg:1)")
              w477 = 1 items=["no exception", "cancel error on match", "set error on match"] ("[exception action] (none:0)")
              n143 = Increment(x=w488) -> (x+1=w487:T6)
              n144 = Enqueue Element(queue=w486, element=w487, error in (no error)=w485) -> (error out=w482:errorcluster)  [unwired: 1 in, 2 out]
              n145 = case shown="True" w483 {
                tunnel: [w489 w493] -> w474
                tunnel: w482 -> [w489 w492]
                tunnel: w484 -> [_ w491]
                frame False {
                }
                frame True {
                  n146 = Unbundle By Name(w491) -> ("LaserCtrlMethod"=w490:T2)
                  n147 = case shown="\"SRS_DG535\"" w490 {
                    tunnel: [w498 w503 w508] -> w493
                    tunnel: w492 -> [w497 w502 w507]
                    tunnel: w491 -> [w495 w501 w506]
                    frame "SDG_II" {
                      n148 = Unbundle By Name(w495) -> ("SDG_ii"=w494:refnum<queue>)
                      n149 = Enqueue Element(queue=w494, element=T11 {"State"=enum."Single Shot", "Parameter"=0.0}, error in (no error)=w497) -> (error out=w498:errorcluster)  [unwired: 1 in, 2 out]
                    }
                    frame "BNC" {
                      n150 = Unbundle By Name(w501) -> ("BNC"=w500:refnum<queue>)
                      n151 = Enqueue Element(queue=w500, element=T12 {"State"=enum."Stop", "Para."=variant}, error in (no error)=w502) -> (error out=w503:errorcluster)  [unwired: 1 in, 2 out]
                    }
                    frame "SRS_DG535" {
                      n152 = Unbundle By Name(w506) -> ("SRS DG535"=w505:refnum<queue>)
                      n153 = Enqueue Element(queue=w505, element=T13 {"State"=enum."Stop", "Para."=variant}, error in (no error)=w507) -> (error out=w508:errorcluster)  [unwired: 1 in, 2 out]
                    }
                  }
                }
              }
              n154 = call <vilib>:"General Error Handler.vi"("type of dialog (OK msg:1)"=w475, "error in (no error)"=w474, "[exception action] (none:0)"=w477, "[exception code]"=1) -> ("error out"=w473:errorcluster)  [unwired: 7 in, 4 out]
            }
            frame "EndOfLine" {
              n155 = Enqueue Element(queue=w521, element=MeanderLoopState."RestoreVelocity", error in (no error)=w520) -> (error out=w517:errorcluster)  [unwired: 1 in, 2 out]
              n156 = Unbundle By Name(w519) -> ("ProcCore_CtrlQueue"=w518:refnum<queue>)
              n157 = Enqueue Element(queue=w518, element=T9 {"Command"=enum."EndOfLine", "Params"=variant}, error in (no error)=w517) -> (error out=w516:errorcluster)  [unwired: 1 in, 2 out]
            }
            frame "CheckPause" {
              n158 = while {
                shift-right: [w536] -> w528
                shift-left: w531 -> [w543]
                tunnel: w530 -> [w544]
                tunnel: [w534] -> w529
                stop <- w540 continue-if-true
                n159 = Preview Queue Element(queue=w544, timeout in ms (-1)=0, error in (no error)=w543) -> (element=w541:T6, timed out?=w538:bool, error out=w537:errorcluster)  [unwired: 1 out]
                n160 = global read "PauseMeander.vi" "Pause Meaner"() -> (w545:bool)
                n161 = Not Equal?(x=MeanderLoopState."Exit", y=w541) -> (x != y?=w539:bool)
                n162 = Compound Arithmetic op=AND(w539, invert w538) -> (w534:bool)
                n163 = Not(x=w534) -> (.not. x?=w533:bool)
                n164 = Or(x=w545, y=w534) -> (x .or. y?=w540:bool)
                n165 = call <userlib>:"Wait (ms)__ogtk.vi"("error in (no error)"=w537, "Wait on Error (FALSE)"=w533, "milliseconds to wait"=u32 200) -> ("error out"=w536:errorcluster)  [unwired: 7 in, 1 out]
              }
            }
            frame "Exit" {
              n166 = Enqueue Element At Opposite End(queue=w547, element=MeanderLoopState."Quit", error in (no error)=w563) -> (queue out=w559:refnum<queue>, error out=w560:errorcluster)  [unwired: 1 in, 1 out]
              n167 = Enqueue Element At Opposite End(queue=w559, element=MeanderLoopState."StopLaser", error in (no error)=w560) -> (queue out=w551:refnum<queue>, error out=w550:errorcluster)  [unwired: 1 in, 1 out]
              n168 = disable-structure shown="Enabled" {
                disable-tunnel: w551 -> [w567 _]
                disable-tunnel: w550 -> [w566 w569]
                disable-tunnel: [w565 w569] -> w549
                frame Disabled {
                  n169 = Enqueue Element At Opposite End(queue=w567, element=MeanderLoopState."EndOfLine", error in (no error)=w566) -> (error out=w565:errorcluster)  [unwired: 1 in, 2 out]
                }
                frame Enabled {
                }
              }
              n170 = Enqueue Element At Opposite End(queue=w562, element=T7 {"State"=enum."STOP", "Params."=variant}, error in (no error)=w549) -> ()  [unwired: 1 in, 3 out]
            }
            frame "RestoreVelocity" {
              n171 = Enqueue Element(queue=w572, element=MeanderLoopState."CheckPause", error in (no error)=w573) -> (error out=w571:errorcluster)  [unwired: 1 in, 2 out]
              n172 = Obtain Queue(name (unnamed)="Status", element data type=T8 {"Position"=[], "Velocity"=[], "Acceleration"=[], "Moving"=FALSE, "Simulation"=FALSE, "tickcount_mov"=0, "tickcount_pos"=0, "NumOfAxis"=0, "Initialized"=FALSE, "CommPort"="", "Range"=[], "Serial Configuration"={"Baud Rate"=0, "Parity"=0, "Data Bits"=0, "Stop Bits"=0, "Flow Control"=0}, "MotorDisabled"=refnum}, error in (no error)=w571) -> (queue out=w586:refnum<queue>, error out=w585:errorcluster)  [unwired: 2 in, 1 out]
              n173 = Bundle By Name(cluster=T7 {"State"=enum."QueryStatus", "Params."=variant} ("element"), "Params."=w586) -> (w587:T7)
              n174 = Dequeue Element(queue=w586, error in (no error)=w585) -> (element=w584:T8, error out=w582:errorcluster)  [unwired: 1 in, 2 out]
              n175 = Enqueue Element(queue=w579, element=w587) -> (queue out=w590:refnum<queue>)  [unwired: 2 in, 2 out]
              n176 = Unbundle By Name(w584) -> ("NumOfAxis"=w583:i32)
              n177 = for {
                N: w583 -> [_]
                tunnel: w590 -> [w595]
                tunnel: w591 -> [w594]
                shift-right: [w592] -> w581
                shift-left: w582 -> [w593]
                i -> [w601]
                n178 = Increment(x=w601) -> (x+1=w599:i32)
                n179 = Bundle By Name(cluster=cluster{"Axis":i32, "Velocity":dbl} {"Axis"=0, "Velocity"=0.0}, "Velocity"=w594, "Axis"=w599) -> (w596:cluster{"Axis":i32, "Velocity":dbl})
                n180 = Bundle By Name(cluster=T7 {"State"=enum."SetVelocity", "Params."=variant} ("element"), "Params."=w596) -> (w598:T7)
                n181 = Enqueue Element(queue=w595, element=w598, error in (no error)=w593) -> (error out=w592:errorcluster)  [unwired: 1 in, 2 out]
              }
            }
            frame "Quit" {
              w602 = TRUE
              # "Dupliate of \"restore high velocity\"\nOtherwise race condition may skip it"
              n182 = Obtain Queue(name (unnamed)="Status", element data type=T8 {"Position"=[], "Velocity"=[], "Acceleration"=[], "Moving"=FALSE, "Simulation"=FALSE, "tickcount_mov"=0, "tickcount_pos"=0, "NumOfAxis"=0, "Initialized"=FALSE, "CommPort"="", "Range"=[], "Serial Configuration"={"Baud Rate"=0, "Parity"=0, "Data Bits"=0, "Stop Bits"=0, "Flow Control"=0}, "MotorDisabled"=refnum}, error in (no error)=w603) -> (queue out=w616:refnum<queue>, error out=w615:errorcluster)  [unwired: 2 in, 1 out]
              n183 = Bundle By Name(cluster=T7 {"State"=enum."QueryStatus", "Params."=variant} ("element"), "Params."=w616) -> (w617:T7)
              n184 = Dequeue Element(queue=w616, error in (no error)=w615) -> (element=w614:T8, error out=w612:errorcluster)  [unwired: 1 in, 2 out]
              n185 = Enqueue Element(queue=w609, element=w617) -> (queue out=w620:refnum<queue>)  [unwired: 2 in, 2 out]
              n186 = Unbundle By Name(w614) -> ("NumOfAxis"=w613:i32)
              n187 = for {
                N: w613 -> [_]
                tunnel: w620 -> [w625]
                tunnel: w621 -> [w624]
                shift-right: [w622] -> w611
                shift-left: w612 -> [w623]
                i -> [w631]
                n188 = Increment(x=w631) -> (x+1=w629:i32)
                n189 = Bundle By Name(cluster=cluster{"Axis":i32, "Velocity":dbl} {"Axis"=0, "Velocity"=0.0}, "Velocity"=w624, "Axis"=w629) -> (w626:cluster{"Axis":i32, "Velocity":dbl})
                n190 = Bundle By Name(cluster=T7 {"State"=enum."SetVelocity", "Params."=variant} ("element"), "Params."=w626) -> (w628:T7)
                n191 = Enqueue Element(queue=w625, element=w628, error in (no error)=w623) -> (error out=w622:errorcluster)  [unwired: 1 in, 2 out]
              }
            }
            frame "Pause" {
              # "Not mature, skip"
              # "Stop stage, laser\nwait\nrestart stage, laser / Quit"
              n192 = while {
                shift-right: [w645] -> w642
                shift-left: w644 -> [w656]
                shift-right: [w647] -> w640
                shift-left: w641 -> [w657]
                stop <- w649 stop-if-true
                n193 = Preview Queue Element(queue=w657, timeout in ms (-1)=0, error in (no error)=w656) -> (queue out=w648:refnum<queue>, element=w654:T6, timed out?=w652:bool, error out=w651:errorcluster)
                n194 = call <userlib>:"Wait (ms)__ogtk.vi"("error in (no error)"=w651, "milliseconds to wait"=u32 200) -> ("error out"=w646:errorcluster)  [unwired: 8 in, 1 out]
                n195 = Equal?(x=T14."Pause", y=w654) -> (x = y?=w653:bool)
                n196 = Compound Arithmetic op=AND(w653, invert w652) -> (w649:bool)
                n197 = case shown="True" w649 {
                  tunnel: w648 -> [w660 w664]
                  tunnel: [w660 w663] -> w647
                  tunnel: w646 -> [w659 w662]
                  tunnel: [w659 w661] -> w645
                  frame False {
                  }
                  frame True {
                    n198 = Dequeue Element(queue=w664, error in (no error)=w662) -> (queue out=w663:refnum<queue>, error out=w661:errorcluster)  [unwired: 1 in, 2 out]
                  }
                }
              }
              n199 = One Button Dialog(message="Internal error. Unexpected pause frame.") -> ()  [unwired: 1 in, 1 out]
              n200 = Enqueue Element At Opposite End(queue=w640, element=MeanderLoopState."StartOfLine", error in (no error)=w642) -> (error out=w643:errorcluster)  [unwired: 1 in, 2 out]
            }
          }
        }
        frame Error {
          n201 = Unbundle By Name(w671) -> ("source"=w670:string)
          n202 = Format Into String(w666) -> (resulting string=w667:string)  [unwired: 3 in, 1 out]
          n203 = Concatenate Strings(w670, w667) -> (w668:string)
          n204 = One Button Dialog(message=w668) -> ()  [unwired: 1 in, 1 out]
        }
      }
      n205 = call <userlib>:"ErrorLog.vi"("error in (no error)"=w86) -> ("error out"=w68:errorcluster)  [unwired: 10 in]
      "Core_iter." <- w73
    }
  }
  "Interupted" <- w39
  n206 = while {
    tunnel: "AppsRef" -> [w682]
    tunnel: w23 -> [w679]
    tunnel: "MotionStageRefs" -> [w678]
    shift-right: [w677] -> w17
    shift-left: FALSE -> [w676]
    stop <- w680 stop-if-true
    # "Interrupted Stop"
    n207 = Dequeue Element(queue=w682) -> (element=w681:T4)  [unwired: 2 in, 3 out]
    n208 = case shown="\"Interrupted_Stop\"" w681 {
      tunnel: [_ FALSE TRUE] -> w680
      tunnel: w679 -> [_ w691 _]
      tunnel: w678 -> [_ w688 _]
      tunnel: [w683 TRUE w693] -> w677
      tunnel: w676 -> [w683 _ w693]
      frame Default {
      }
      frame "Interrupted_Stop" {
        n209 = Enqueue Element At Opposite End(queue=w691, element=MeanderLoopState."Exit", timeout in ms (-1)=1000) -> (timed out?=→"timed out?":bool, error out=w686:errorcluster)  [unwired: 1 in, 1 out]
        n210 = Enqueue Element At Opposite End(queue=w688, element=T7 {"State"=enum."STOP", "Params."=variant}, error in (no error)=w686) -> ()  [unwired: 1 in, 3 out]
      }
      frame "Quit_SubProgram" {
      }
    }
  }
  n211 = Increment(x=w42) -> (x+1=→"Scanned Lines":i32)
  n212 = Unbundle By Name(w31) -> ("Feedback"=w30:refnum<queue>, "InfoRef"=w41:refnum<vi>)
  n213 = Release Queue "Only CoreLoop need it"(queue=w30, error in (no error)=w29) -> (error out=w28:errorcluster)  [unwired: 1 in, 2 out]
  n214 = property class="Str"(reference=w41, error in=w28, "Value"="") -> (error out=w32:errorcluster)  [unwired: 1 out]
  n215 = Release Queue(queue=w23, error in (no error)=w32) -> (error out=w20:errorcluster)  [unwired: 1 in, 2 out]
  n216 = Enqueue Element(queue="AppsRef", element=States-AToF."Quit_SubProgram", error in (no error)=w20) -> (error out=w18:errorcluster)  [unwired: 1 in, 2 out]
  n217 = case shown="True" w17 {
    tunnel: w18 -> [_ w695]
    tunnel: w10 -> [_ w698]
    frame False {
    }
    frame True {
      n218 = Generate User Event(user event=w698, event data cluster=cluster{"Quit":bool} {"Quit"=TRUE} ("event data"), error in=w695) -> (error out=w696:errorcluster)  [unwired: 1 in, 1 out]
      n219 = call <vilib>:"Clear Errors.vi"("error in (no error)"=w696) -> ()  [unwired: 6 in, 1 out]
    }
  }
  n220 = Enqueue Element At Opposite End(queue="AppsRef", element=States-AToF."Interrupted_Stop", timeout in ms (-1)=1000, error in (no error)=w8) -> (error out=w27:errorcluster)  [unwired: 2 out]
  n221 = call <vilib>:"Clear Errors.vi"("error in (no error)"=w27) -> ("error out"=w21:errorcluster)  [unwired: 6 in]
  n222 = Merge Errors(w21, w18) -> (w19:errorcluster)
  n223 = Release Queue(queue=w16, error in (no error)=w19) -> (error out=→"error out":errorcluster)  [unwired: 1 in, 2 out]
